vi "sequencing.vi"() -> ()   [LabVIEW 2023]
uses:
  <vilib>/numeric/Random Number (Range) DBL.vi
panel:
  out "Numeric 2":i32
  out "Numeric":i32
  out "number 2":dbl
  out "Waveform Chart 2":dbl(graph)
  out "Waveform Chart":dbl(graph)
  in  "stop":bool
  out "number":dbl
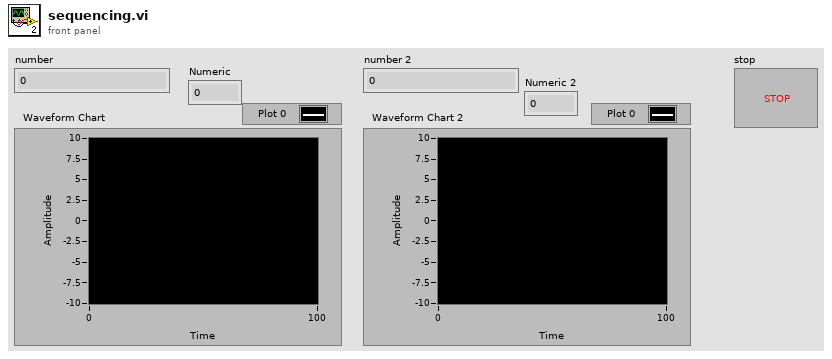
[diagram p1: front panel]
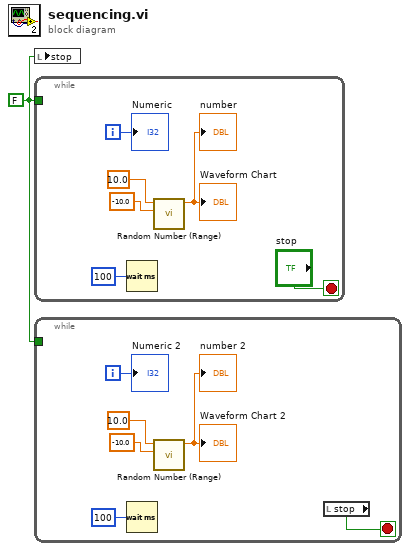
[diagram p0: block diagram]
diagram:
  w1 = FALSE ("stop")
  n1 = local write "stop"(w1) -> ()
  n2 = while {
    tunnel: w1 -> [_]
    i -> [w2]
    stop <- "stop" stop-if-true
    n3 = Wait (ms)(milliseconds to wait=u32 100) -> ()  [unwired: 1 out]
    n4 = call-poly <vilib>:"Random Number (Range).vi"("lower bound (0)"=-10.0, "upper bound (100)"=10.0) -> ("number"=→"number" →"Waveform Chart":dbl)  [unwired: 9 in]
    "Numeric" <- w2
  }
  n5 = while {
    tunnel: w1 -> [_]
    i -> [w9]
    stop <- w8 stop-if-true
    n6 = Wait (ms)(milliseconds to wait=u32 100) -> ()  [unwired: 1 out]
    n7 = call-poly <vilib>:"Random Number (Range).vi"("lower bound (0)"=-10.0, "upper bound (100)"=10.0) -> ("number"=→"number 2" →"Waveform Chart 2":dbl)  [unwired: 9 in]
    n8 = local read "stop"() -> (w8:bool)
    "Numeric 2" <- w9
  }
